vi "update_zc_info6-cz.vi"(0 "ywxinxi":string, 6 "number":string, 7 "status":string, 8 "syren":string, 9 "zrren":string, 10 "zrbumen":string) -> (1 "data_str":string)   [LabVIEW 2017, in "Lib_code.lvlib"]
uses:
  Lib_code.lvlib
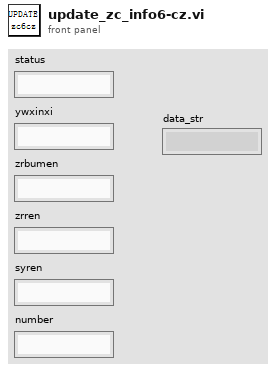
[diagram p1: front panel]
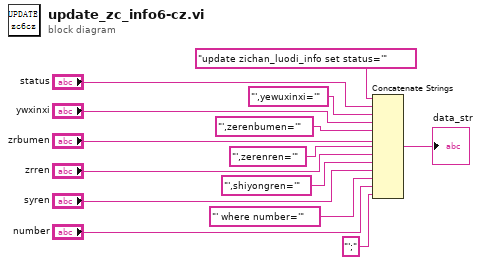
[diagram p0: block diagram]
diagram:
  n1 = Concatenate Strings("update zichan_luodi_info set status='" ("Command Text"), "status", "',yewuxinxi='" ("字符串"), "ywxinxi", "',zerenbumen='" ("字符串"), "zrbumen", "',zerenren='" ("字符串"), "zrren", "',shiyongren='" ("字符串"), "syren", "' where number='" ("字符串"), "number", "';" ("字符串")) -> (→"data_str":string)
